vi "Symphony DatSock_Read.vi"() -> ()   [LabVIEW 2019]
panel:
  out "timestamp":timestamp
  out "Tableau":dbl[][](array[numeric])
  in  "stop":bool
  in  "URL":string
  in  "entrée d'erreur (pas d'erreur)":errorcluster
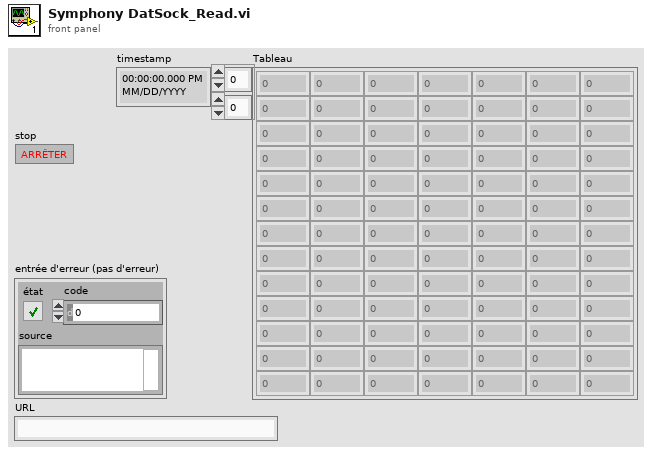
[diagram p1: front panel]
types:
  T1 = enum16{"Read", "Write", "ReadWrite", "BufferedRead", "BufferedReadWrite"}
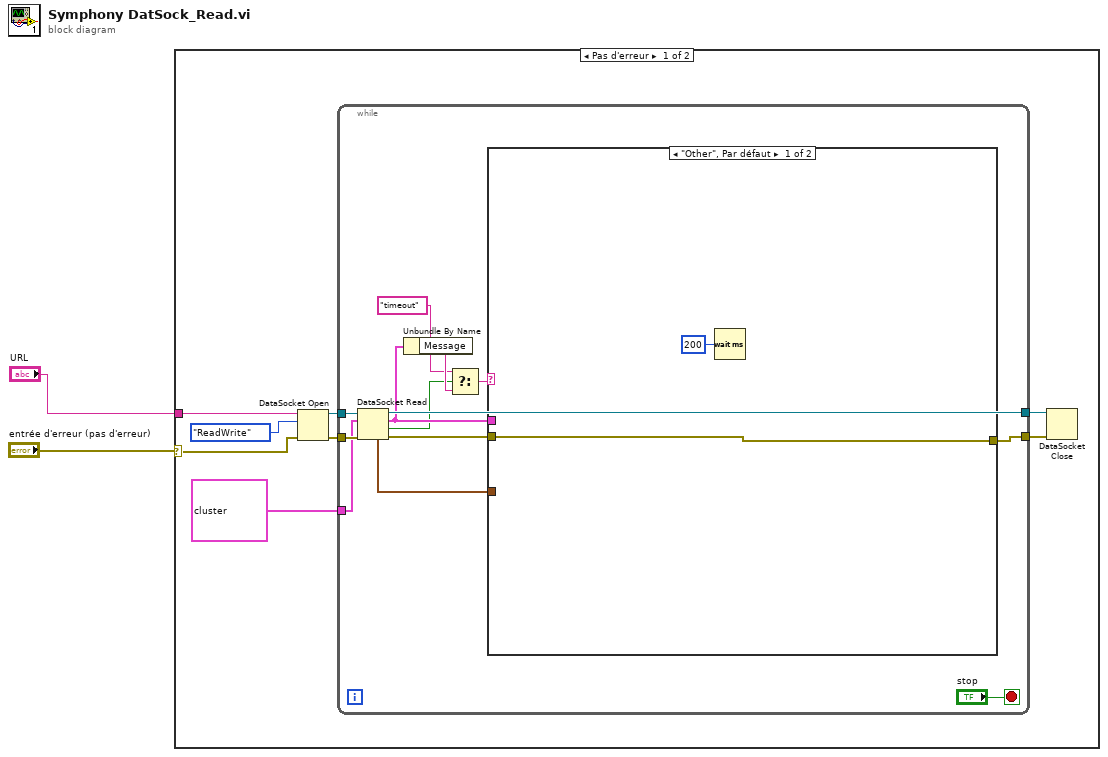
[diagram p0: block diagram]
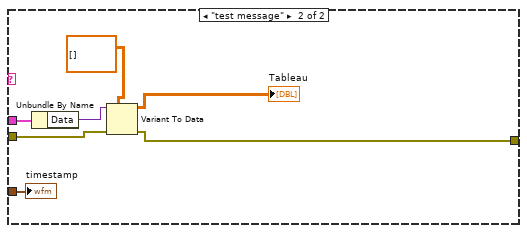
[diagram p2: hidden frame]
diagram:
  n1 = case shown="Pas d'erreur" "entrée d'erreur (pas d'erreur)" {
    selector: "entrée d'erreur (pas d'erreur)" -> [w9 _]
    tunnel: "URL" -> [w10 _]
    frame No Error {
      n2 = DataSocket Open(8:w9, 10:T1."ReadWrite" ("mode"), 11:w10) -> (0:w7:errorcluster, 3:w5:refnum<k13>)  [unwired: 1 in]
      n3 = while {
        tunnel: w7 -> [w23]
        tunnel: cluster{"Message":string, "Data":variant, i32} {"Message"="NoMessage", "Data"=variant, 0} ("élément") -> [w22]
        tunnel: w5 -> [w21]
        tunnel: [w17] -> w4
        tunnel: [w20] -> w3
        stop <- "stop" stop-if-true
        n4 = DataSocket Read(8:w23, 10:w22, 11:w21) -> (0:w16:errorcluster, 1:w11:bool, 2:w18:cluster{"Message":string, "Data":variant, i32}, 3:w20:refnum<k13>, 4:w15:timestamp)  [unwired: 2 in, 2 out]
        n5 = Unbundle By Name(w18) -> ("Message"=w13:string)
        n6 = Select(t="timeout" ("cas vrai"), s=w11, f=w13) -> (s? t:f=w14:string)
        n7 = case shown="\"Other\", Par défaut" w14 {
          tunnel: w18 -> [_ w32]
          tunnel: [w25 w27] -> w17
          tunnel: w16 -> [w25 w28]
          tunnel: w15 -> [_ w26]
          frame "Other", Default {
            n8 = Wait (ms)(milliseconds to wait=u32 200 ("attente (ms)")) -> ()  [unwired: 1 out]
          }
          frame "test message" {
            n9 = Unbundle By Name(w32) -> ("Data"=w29:variant)
            n10 = Variant To Data(error in=w28, type=dbl[][] [] ("Tableau"), Variant=w29) -> (data=→"Tableau":dbl[][], error out=w27:errorcluster)
            "timestamp" <- w26
          }
        }
      }
      n11 = DataSocket Close(8:w4, 11:w3) -> ()  [unwired: 1 in, 2 out]
    }
    frame Error {
    }
  }
